vi "Manage Error.vi"(0 "VI in Error":refnum<vi>, 7 "Code Erreur":T1, 9 "Text":string, 11 "error in (no error)":errorcluster caption="entrée d'erreur (pas d'erreur)") -> (8 "error out":errorcluster caption="sortie d'erreur")   [LabVIEW 2020, in "Library Commun.lvlib"]
uses:
  Library Commun.lvlib
  TypeDef/Liste Error.ctl
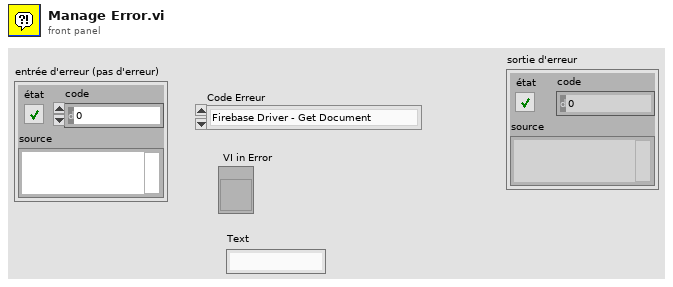
[diagram p1: front panel]
types:
  T1 = typedef "Library Commun.lvlib/Liste Error.ctl" = enum16{"Firebase Driver - Get Document", "Firebase Driver - Get Document With Where", "Firebase Driver - Delete Document", "Firebase Driver - Set Document", "Firebase Driver - Update Document", "Firebase Altyor - Search Document Bench", "Firebase Altyor - Class Not in Firebase", "Spectrum_Analyser - Timeout", "Relay Board - Qty Relay", "DIO - Pb Funtion", "Power_Supply - Peripherical not find", "Mutimeter - Peripherical not find", "Instrument - Function Not Used", "Instrument - Instrument name not specified", "Instrument - Allready Initialised", "Instrument - TimeOut", "Instrument - the instrument must be Initialise before", "Instrument - Frame Not received", "Instrument - Frame Nok", "Test - Initialise the File_for_Save", "Test - Timeout", "Test - Cmd Error", "FGV - Variable ", "BDD FireBase - Define Class", "SN - Class Not Define"}
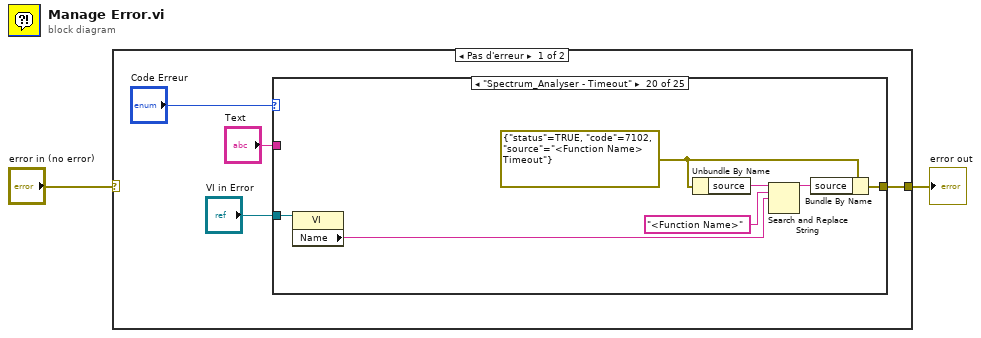
[diagram p0: block diagram]
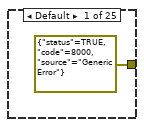
[diagram p2: hidden frame]
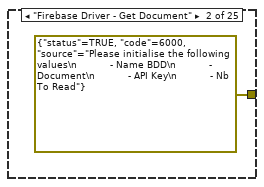
[diagram p3: hidden frame]
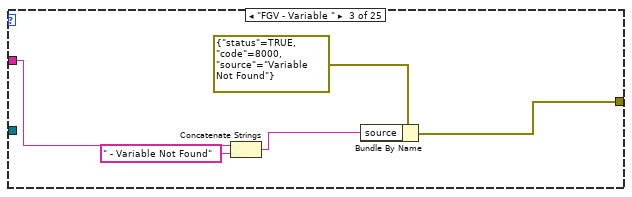
[diagram p4: hidden frame]
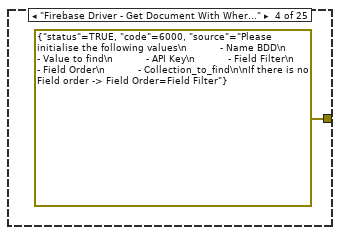
[diagram p5: hidden frame]
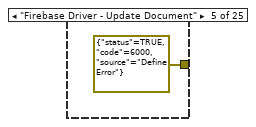
[diagram p6: hidden frame]
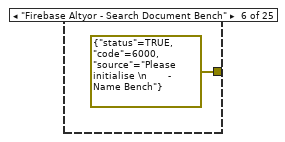
[diagram p7: hidden frame]
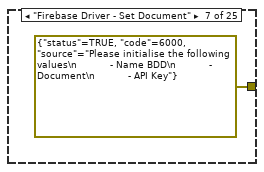
[diagram p8: hidden frame]
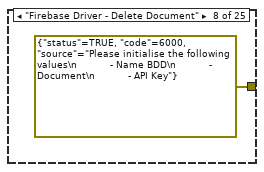
[diagram p9: hidden frame]
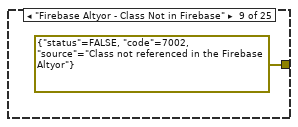
[diagram p10: hidden frame]
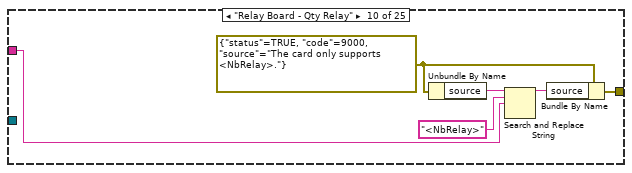
[diagram p11: hidden frame]
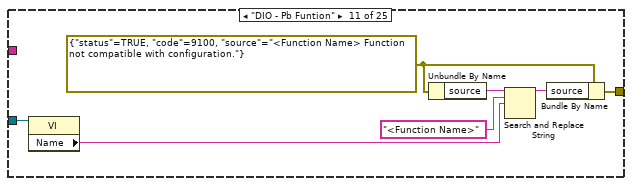
[diagram p12: hidden frame]
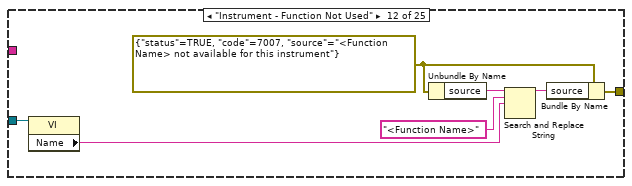
[diagram p13: hidden frame]
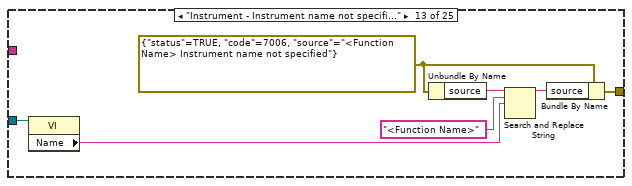
[diagram p14: hidden frame]
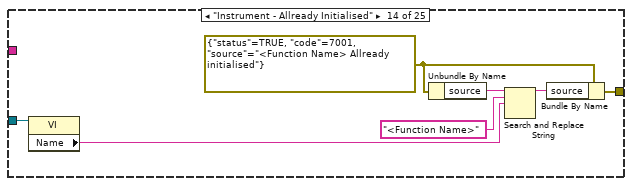
[diagram p15: hidden frame]
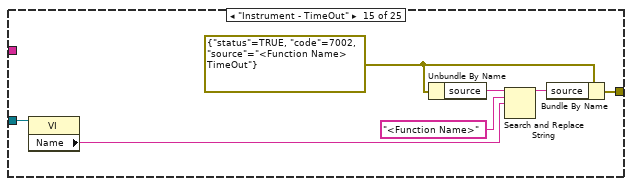
[diagram p16: hidden frame]
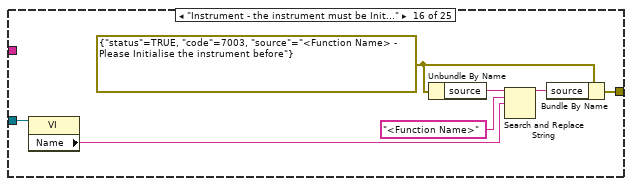
[diagram p17: hidden frame]
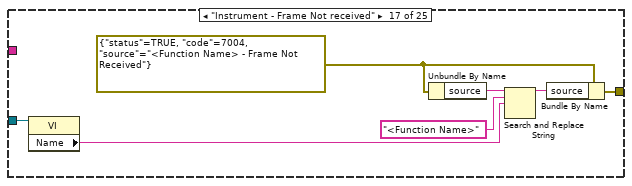
[diagram p18: hidden frame]
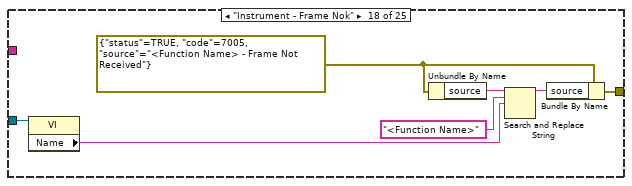
[diagram p19: hidden frame]
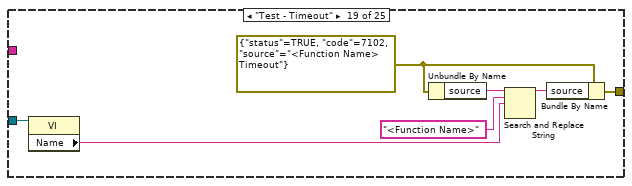
[diagram p20: hidden frame]
diagram:
  n1 = case shown="Pas d'erreur" "error in (no error)" {
    selector: "error in (no error)" -> [_ w131]
    tunnel: [w3 w131] -> w2
    frame No Error {
      n2 = case shown="\"Spectrum_Analyser - Timeout\"" "Code Erreur" {
        tunnel: [errorcluster {"status"=TRUE, "code"=8000, "source"="Generic Error"} ("cas vrai") errorcluster {"status"=TRUE, "code"=6000, "source"="Please initialise the following values\n           - Name BDD\n           - Document\n           - API Key\n           - Nb To Read"} ("cas vrai") w10 errorcluster {"status"=TRUE, "code"=6000, "source"="Please initialise the following values\n           - Name BDD\n           - Value to find\n           - API Key\n           - Field Filter\n           - Field Order\n           - Collection_to_find\n\nIf there is no Field order -> Field Order=Field Filter"} ("cas vrai") errorcluster {"status"=TRUE, "code"=6000, "source"="Define Error"} ("cas vrai") errorcluster {"status"=TRUE, "code"=6000, "source"="Please initialise \n       - Name Bench"} ("cas vrai") errorcluster {"status"=TRUE, "code"=6000, "source"="Please initialise the following values\n           - Name BDD\n           - Document\n           - API Key"} ("cas vrai") errorcluster {"status"=TRUE, "code"=6000, "source"="Please initialise the following values\n           - Name BDD\n           - Document\n           - API Key"} ("cas vrai") errorcluster {"status"=FALSE, "code"=7002, "source"="Class not referenced in the Firebase Altyor"} ("error out") w21 w28 w39 w41 w48 w55 w63 w70 w77 w83 w90 w98 w105 w112 w119 w126] -> w3
        tunnel: "VI in Error" -> [_ _ _ _ _ _ _ _ _ _ w27 w38 w42 w47 w54 w62 w69 w76 w84 w91 w97 w104 w111 w118 w125]
        tunnel: "Text" -> [_ _ w13 _ _ _ _ _ _ w20 _ _ _ _ _ _ _ _ _ _ _ _ _ _ _]
        frame Default {
        }
        frame "Firebase Driver - Get Document" {
        }
        frame "FGV - Variable " {
          n3 = Concatenate Strings(w13, " - Variable Not Found" ("chaîne")) -> (w9:string)
          n4 = Bundle By Name(cluster=errorcluster {"status"=TRUE, "code"=8000, "source"="Variable Not Found"} ("cas vrai"), "source"=w9) -> (w10:errorcluster)
        }
        frame "Firebase Driver - Get Document With Where" {
        }
        frame "Firebase Driver - Update Document" {
        }
        frame "Firebase Altyor - Search Document Bench" {
        }
        frame "Firebase Driver - Set Document" {
        }
        frame "Firebase Driver - Delete Document" {
        }
        frame "Firebase Altyor - Class Not in Firebase" {
        }
        frame "Relay Board - Qty Relay" {
          w22 = errorcluster {"status"=TRUE, "code"=9000, "source"="The card only supports <NbRelay>."} ("cas vrai")
          n5 = Unbundle By Name(w22) -> ("source"=w25:string)
          n6 = Search and Replace String(input string=w25, search string="<NbRelay>" ("chaîne recherchée"), replace string=w20) -> (result string=w23:string)  [unwired: 5 in, 3 out]
          n7 = Bundle By Name(cluster=w22, "source"=w23) -> (w21:errorcluster)
        }
        frame "DIO - Pb Funtion" {
          w29 = errorcluster {"status"=TRUE, "code"=9100, "source"="<Function Name> Function not compatible with configuration."} ("cas vrai")
          n8 = property class="VI"(reference=w27) -> ("Name"=w26:string)  [unwired: 1 in, 2 out]
          n9 = Unbundle By Name(w29) -> ("source"=w32:string)
          n10 = Search and Replace String(input string=w32, search string="<Function Name>" ("chaîne recherchée"), replace string=w26) -> (result string=w30:string)  [unwired: 5 in, 3 out]
          n11 = Bundle By Name(cluster=w29, "source"=w30) -> (w28:errorcluster)
        }
        frame "Instrument - Function Not Used" {
          w34 = errorcluster {"status"=TRUE, "code"=7007, "source"="<Function Name> not available for this instrument"} ("error IO")
          n12 = property class="VI"(reference=w38) -> ("Name"=w33:string)  [unwired: 1 in, 2 out]
          n13 = Unbundle By Name(w34) -> ("source"=w37:string)
          n14 = Search and Replace String(input string=w37, search string="<Function Name>" ("chaîne recherchée"), replace string=w33) -> (result string=w35:string)  [unwired: 5 in, 3 out]
          n15 = Bundle By Name(cluster=w34, "source"=w35) -> (w39:errorcluster)
        }
        frame "Instrument - Instrument name not specified" {
          w40 = errorcluster {"status"=TRUE, "code"=7006, "source"="<Function Name> Instrument name not specified"} ("error IO")
          n16 = property class="VI"(reference=w42) -> ("Name"=w44:string)  [unwired: 1 in, 2 out]
          n17 = Unbundle By Name(w40) -> ("source"=w46:string)
          n18 = Search and Replace String(input string=w46, search string="<Function Name>" ("chaîne recherchée"), replace string=w44) -> (result string=w45:string)  [unwired: 5 in, 3 out]
          n19 = Bundle By Name(cluster=w40, "source"=w45) -> (w41:errorcluster)
        }
        frame "Instrument - Allready Initialised" {
          w50 = errorcluster {"status"=TRUE, "code"=7001, "source"="<Function Name> Allready initialised"} ("error IO")
          n20 = property class="VI"(reference=w47) -> ("Name"=w49:string)  [unwired: 1 in, 2 out]
          n21 = Unbundle By Name(w50) -> ("source"=w53:string)
          n22 = Search and Replace String(input string=w53, search string="<Function Name>" ("chaîne recherchée"), replace string=w49) -> (result string=w51:string)  [unwired: 5 in, 3 out]
          n23 = Bundle By Name(cluster=w50, "source"=w51) -> (w48:errorcluster)
        }
        frame "Instrument - TimeOut" {
          w57 = errorcluster {"status"=TRUE, "code"=7002, "source"="<Function Name> TimeOut"} ("error IO")
          n24 = property class="VI"(reference=w54) -> ("Name"=w56:string)  [unwired: 1 in, 2 out]
          n25 = Unbundle By Name(w57) -> ("source"=w60:string)
          n26 = Search and Replace String(input string=w60, search string="<Function Name>" ("chaîne recherchée"), replace string=w56) -> (result string=w58:string)  [unwired: 5 in, 3 out]
          n27 = Bundle By Name(cluster=w57, "source"=w58) -> (w55:errorcluster)
        }
        frame "Instrument - the instrument must be Initialise before" {
          w61 = errorcluster {"status"=TRUE, "code"=7003, "source"="<Function Name> - Please Initialise the instrument before"} ("cas faux")
          n28 = property class="VI"(reference=w62) -> ("Name"=w64:string)  [unwired: 1 in, 2 out]
          n29 = Unbundle By Name(w61) -> ("source"=w67:string)
          n30 = Search and Replace String(input string=w67, search string="<Function Name>" ("chaîne recherchée"), replace string=w64) -> (result string=w65:string)  [unwired: 5 in, 3 out]
          n31 = Bundle By Name(cluster=w61, "source"=w65) -> (w63:errorcluster)
        }
        frame "Instrument - Frame Not received" {
          w68 = errorcluster {"status"=TRUE, "code"=7004, "source"="<Function Name> - Frame Not Received"} ("cas faux")
          n32 = property class="VI"(reference=w69) -> ("Name"=w71:string)  [unwired: 1 in, 2 out]
          n33 = Unbundle By Name(w68) -> ("source"=w74:string)
          n34 = Search and Replace String(input string=w74, search string="<Function Name>" ("chaîne recherchée"), replace string=w71) -> (result string=w72:string)  [unwired: 5 in, 3 out]
          n35 = Bundle By Name(cluster=w68, "source"=w72) -> (w70:errorcluster)
        }
        frame "Instrument - Frame Nok" {
          w75 = errorcluster {"status"=TRUE, "code"=7005, "source"="<Function Name> - Frame Not Received"} ("cas faux")
          n36 = property class="VI"(reference=w76) -> ("Name"=w78:string)  [unwired: 1 in, 2 out]
          n37 = Unbundle By Name(w75) -> ("source"=w81:string)
          n38 = Search and Replace String(input string=w81, search string="<Function Name>" ("chaîne recherchée"), replace string=w78) -> (result string=w79:string)  [unwired: 5 in, 3 out]
          n39 = Bundle By Name(cluster=w75, "source"=w79) -> (w77:errorcluster)
        }
        frame "Test - Timeout" {
          w82 = errorcluster {"status"=TRUE, "code"=7102, "source"="<Function Name> Timeout"} ("error IO")
          n40 = property class="VI"(reference=w84) -> ("Name"=w86:string)  [unwired: 1 in, 2 out]
          n41 = Unbundle By Name(w82) -> ("source"=w88:string)
          n42 = Search and Replace String(input string=w88, search string="<Function Name>" ("chaîne recherchée"), replace string=w86) -> (result string=w87:string)  [unwired: 5 in, 3 out]
          n43 = Bundle By Name(cluster=w82, "source"=w87) -> (w83:errorcluster)
        }
        frame "Spectrum_Analyser - Timeout" {
          w89 = errorcluster {"status"=TRUE, "code"=7102, "source"="<Function Name> Timeout"} ("error IO")
          n44 = property class="VI"(reference=w91) -> ("Name"=w93:string)  [unwired: 1 in, 2 out]
          n45 = Unbundle By Name(w89) -> ("source"=w95:string)
          n46 = Search and Replace String(input string=w95, search string="<Function Name>" ("chaîne recherchée"), replace string=w93) -> (result string=w94:string)  [unwired: 5 in, 3 out]
          n47 = Bundle By Name(cluster=w89, "source"=w94) -> (w90:errorcluster)
        }
        frame "Test - Initialise the File_for_Save" {
          w96 = errorcluster {"status"=TRUE, "code"=7101, "source"="<Function Name> - Please Initialise File_For_ Save"} ("cas faux")
          n48 = property class="VI"(reference=w97) -> ("Name"=w99:string)  [unwired: 1 in, 2 out]
          n49 = Unbundle By Name(w96) -> ("source"=w102:string)
          n50 = Search and Replace String(input string=w102, search string="<Function Name>" ("chaîne recherchée"), replace string=w99) -> (result string=w100:string)  [unwired: 5 in, 3 out]
          n51 = Bundle By Name(cluster=w96, "source"=w100) -> (w98:errorcluster)
        }
        frame "Test - Cmd Error" {
          w103 = errorcluster {"status"=TRUE, "code"=7101, "source"="<Function Name> - Error on Command"} ("cas faux")
          n52 = property class="VI"(reference=w104) -> ("Name"=w106:string)  [unwired: 1 in, 2 out]
          n53 = Unbundle By Name(w103) -> ("source"=w109:string)
          n54 = Search and Replace String(input string=w109, search string="<Function Name>" ("chaîne recherchée"), replace string=w106) -> (result string=w107:string)  [unwired: 5 in, 3 out]
          n55 = Bundle By Name(cluster=w103, "source"=w107) -> (w105:errorcluster)
        }
        frame "Power_Supply - Peripherical not find" {
          w110 = errorcluster {"status"=TRUE, "code"=7201, "source"="<Function Name> - Please Connect the Power-supply"} ("cas faux")
          n56 = property class="VI"(reference=w111) -> ("Name"=w113:string)  [unwired: 1 in, 2 out]
          n57 = Unbundle By Name(w110) -> ("source"=w116:string)
          n58 = Search and Replace String(input string=w116, search string="<Function Name>" ("chaîne recherchée"), replace string=w113) -> (result string=w114:string)  [unwired: 5 in, 3 out]
          n59 = Bundle By Name(cluster=w110, "source"=w114) -> (w112:errorcluster)
        }
        frame "Mutimeter - Peripherical not find" {
          w117 = errorcluster {"status"=TRUE, "code"=7201, "source"="<Function Name> - Please Connect the Multimeter"} ("cas faux")
          n60 = property class="VI"(reference=w118) -> ("Name"=w120:string)  [unwired: 1 in, 2 out]
          n61 = Unbundle By Name(w117) -> ("source"=w123:string)
          n62 = Search and Replace String(input string=w123, search string="<Function Name>" ("chaîne recherchée"), replace string=w120) -> (result string=w121:string)  [unwired: 5 in, 3 out]
          n63 = Bundle By Name(cluster=w117, "source"=w121) -> (w119:errorcluster)
        }
        frame "BDD FireBase - Define Class" {
          w124 = errorcluster {"status"=TRUE, "code"=6000, "source"="Plz Define Class in <Function Name>"} ("cas faux")
          n64 = property class="VI"(reference=w125) -> ("Name"=w127:string)  [unwired: 1 in, 2 out]
          n65 = Unbundle By Name(w124) -> ("source"=w130:string)
          n66 = Search and Replace String(input string=w130, search string="<Function Name>" ("chaîne recherchée"), replace string=w127) -> (result string=w128:string)  [unwired: 5 in, 3 out]
          n67 = Bundle By Name(cluster=w124, "source"=w128) -> (w126:errorcluster)
        }
      }
    }
    frame Error {
    }
  }
  "error out" <- w2
